vi "buildPath.vi"() -> (3 "String":string)   [LabVIEW 2013]
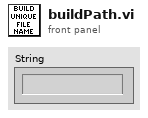
[diagram p1: front panel]
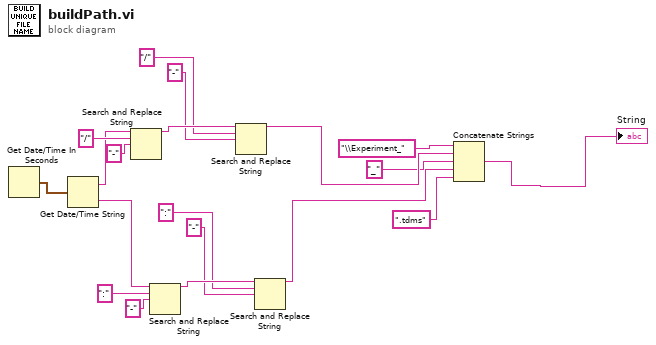
[diagram p0: block diagram]
diagram:
  n1 = Get Date/Time In Seconds() -> (seconds since 1Jan1904=w1:timestamp)
  n2 = Get Date/Time String(seconds (now)=w1) -> (date string=w6:string, time string=w18:string)  [unwired: 2 in]
  n3 = Search and Replace String(input string=w6, search string="/", replace string="-" ("replace string (\"\")")) -> (result string=w11:string)  [unwired: 5 in, 3 out]
  n4 = Search and Replace String(input string=w18, search string=":", replace string="-" ("replace string (\"\")")) -> (result string=w17:string)  [unwired: 5 in, 3 out]
  n5 = Search and Replace String(input string=w11, search string="/", replace string="-" ("replace string (\"\")")) -> (result string=w12:string)  [unwired: 5 in, 3 out]
  n6 = Search and Replace String(input string=w17, search string=":", replace string="-" ("replace string (\"\")")) -> (result string=w19:string)  [unwired: 5 in, 3 out]
  n7 = Concatenate Strings("\\Experiment_" ("string"), w12, "_" ("string"), w19, ".tdms" ("string")) -> (→"String":string)
